vi "Set APU.vi"(8 "error in (no error)":errorcluster, 10 "APU Settings":T1 {"des accel" min=0.0 format="%#_p"}, 11 "APU in":refnum<k24>) -> (0 "error out":errorcluster, 3 "APU out":refnum<k24>)   [LabVIEW 2020, in "Engine Simulation Toolkit Scripting API.lvlib"]
uses:
  Engine Simulation Toolkit Scripting API.lvlib
  NationalInstruments.VeriStand.SystemDefinitionAPI
  APU Settings.ctl
  Shared/Constants and GUIDs.vi
  Shared/Properties.vi
  <vilib>/NI VeriStand/Custom Device API/Set Item Property (Double).vi
  <vilib>/NI VeriStand/Custom Device Tools/Custom Device Utility Library/NI VeriStand - Search for Item by Name.vi
  <vilib>/NI VeriStand/Custom Device API/Set Item Property (Boolean).vi
  <vilib>/NI VeriStand/Custom Device API/Custom Device API.lvlib
  Shared/Engine Simulation Toolkit Shared.lvlib
  <vilib>/NI VeriStand/Custom Device Tools/Custom Device Utility Library/Custom Device Utility Library.lvlib
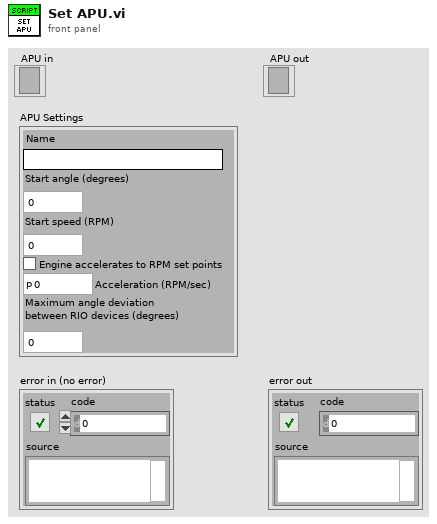
[diagram p1: front panel]
types:
  T1 = typedef "Engine Simulation Toolkit Scripting API.lvlib/APU Settings.ctl" = cluster{"Name":string, "Start angle (degrees)":dbl, "des speed":dbl, "Acceleration":bool, "des accel":dbl, "Maximum angle deviation\nbetween RIO devices (degrees)":dbl}
  T2 = typedef "Engine Simulation Toolkit Shared.lvlib/Channel.ctl" = cluster{"Name":string, "Units":string, "Default":dbl, "Description":string, "Scalable":bool}
  T3 = typedef "Custom Device API.lvlib/Custom Device Item Ref.ctl" = u64
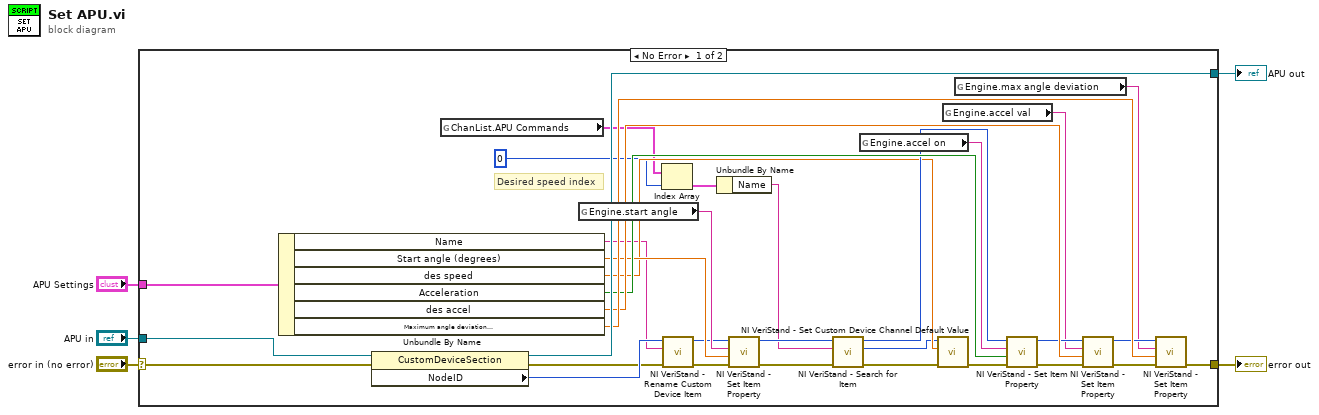
[diagram p0: block diagram]
diagram:
  n1 = case shown="No Error" "error in (no error)" {
    selector: "error in (no error)" -> [w38 w40]
    tunnel: [w37 w40] -> w4
    tunnel: [w36 w39] -> w3
    tunnel: "APU in" -> [w35 w39]
    tunnel: "APU Settings" -> [w34 _]
    frame No Error {
      # "Desired speed index"
      n2 = Unbundle By Name(w34) -> ("Name"=w6:string, "Start angle (degrees)"=w21:dbl, "des speed"=w17:dbl, "Acceleration"=w25:bool, "des accel"=w29:dbl, "Maximum angle deviation\nbetween RIO devices (degrees)"=w33:dbl)
      n3 = property class="CustomDeviceSection"(reference=w35, error in=w38) -> (reference out=w36:refnum<k24>, error out=w9:errorcluster, "NodeID"=w10:u64)
      n4 = global read "Constants and GUIDs.vi" "ChanList.APU Commands"() -> (w11:T2[])
      n5 = global read "Properties.vi" "Engine.start angle"() -> (w18:string)
      n6 = Index Array(array=w11, index=0) -> (element=w12:T2)
      n7 = call <vilib>:"NI VeriStand - Rename Custom Device Item.vi"("error in (no error)"=w9, "New Name"=w6, "Item Ref in"=w10) -> ("error out"=w8:errorcluster, "Item Ref out"=w7:T3)  [unwired: 6 in, 1 out]
      n8 = Unbundle By Name(w12) -> ("Name"=w15:string)
      n9 = call-poly <vilib>:"NI VeriStand - Set Item Property.vi"("error in (no error)"=w8, "Value"=w21, "Property Name"=w18, "Item Ref in"=w7) -> ("error out"=w19:errorcluster, "Item Ref out"=w20:T3)  [unwired: 5 in, 1 out]
      n10 = call-poly <vilib>:"NI VeriStand - Search for Item.vi"("error in"=w19, "Item Name"=w15, "Section Ref in"=w20) -> ("error out"=w14:errorcluster, "Item Ref"=w16:T3, "Section Ref out"=w23:T3)  [unwired: 5 in, 1 out]
      n11 = global read "Properties.vi" "Engine.accel on"() -> (w22:string)
      n12 = call <vilib>:"NI VeriStand - Set Custom Device Channel Default Value.vi"("error in (no error)"=w14, "Default Value"=w17, "Channel Ref in"=w16) -> ("error out"=w24:errorcluster)  [unwired: 7 in, 1 out]
      n13 = global read "Properties.vi" "Engine.accel val"() -> (w26:string)
      n14 = global read "Properties.vi" "Engine.max angle deviation"() -> (w30:string)
      n15 = call-poly <vilib>:"NI VeriStand - Set Item Property.vi"("error in (no error)"=w24, "Value"=w25, "Property Name"=w22, "Item Ref in"=w23) -> ("error out"=w28:errorcluster, "Item Ref out"=w27:T3)  [unwired: 5 in, 1 out]
      n16 = call-poly <vilib>:"NI VeriStand - Set Item Property.vi"("error in (no error)"=w28, "Value"=w29, "Property Name"=w26, "Item Ref in"=w27) -> ("error out"=w31:errorcluster, "Item Ref out"=w32:T3)  [unwired: 5 in, 1 out]
      n17 = call-poly <vilib>:"NI VeriStand - Set Item Property.vi"("error in (no error)"=w31, "Value"=w33, "Property Name"=w30, "Item Ref in"=w32) -> ("error out"=w37:errorcluster)  [unwired: 5 in, 2 out]
    }
    frame Error {
    }
  }
  "error out" <- w4
  "APU out" <- w3
